vi "PreSequenceAcquisition.vi"(8 "error in (no error)":errorcluster, 10 "Acquisition Params":T1 {"Interval" min=0.0 max=99999.0; "Frames" min=0.0 max=5000.0; "ExposureMs" min=0.0 max=99999.0}, 11 "Camera_Prime95B in":refnum<class "Camera_Prime95B.lvclass">) -> (0 "error out":errorcluster, 3 "Camera_Prime95B out":refnum<class "Camera_Prime95B.lvclass">)   [LabVIEW 2020, in "Camera_Prime95B.lvlib" / "Camera_Prime95B.lvclass"]
uses:
  Camera_Prime95B.lvclass
  Acquisition Params.ctl
  Camera_Prime95B.lvclass/Camera_Prime95B.ctl
  D:/Daguan/Development/MMicroscopyAF/Model/Real Hardware/Camera_Prime95B/Camera_Prime95B/Dependencies/PVCamNET.dll
  Dependencies/PVCamNET.dll
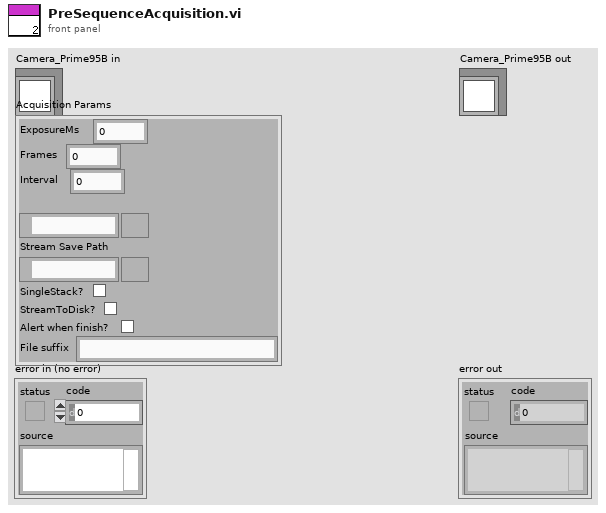
[diagram p1: front panel]
types:
  T1 = typedef "Camera_Prime95B.lvlib/Camera_Prime95B.lvclass/Acquisition Params.ctl" = cluster{"ExposureMs":dbl, "Frames":dbl, "Interval":dbl, "Save Path":path, "Stream Save Path":path, "SingleStack?":bool, "StreamToDisk?":bool, "Alert when finish?":bool, "File suffix":string}
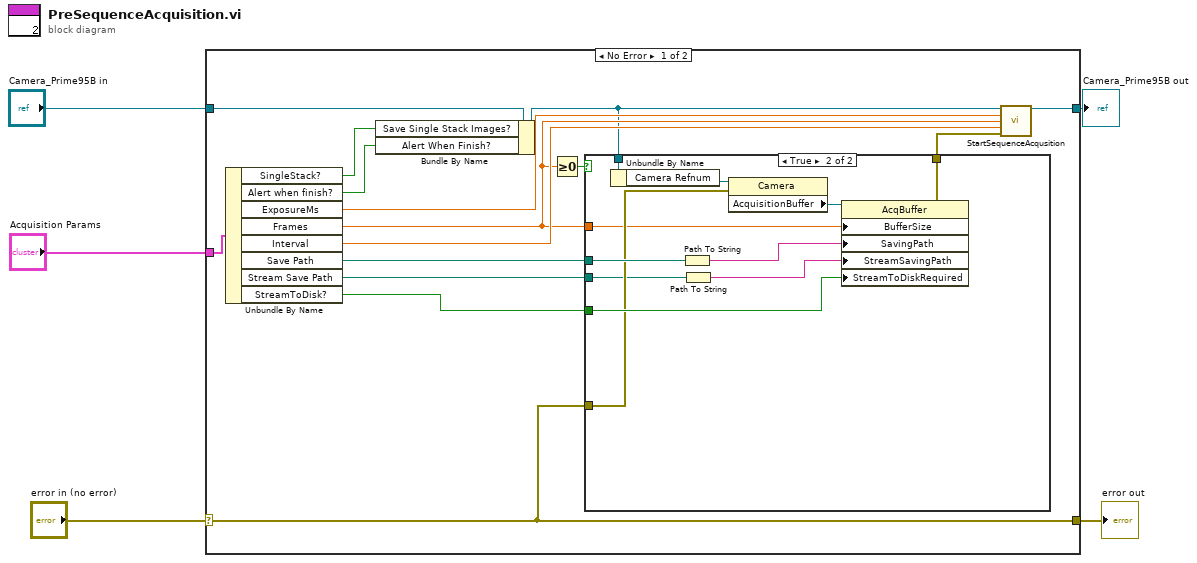
[diagram p0: block diagram]
diagram:
  n1 = case shown="No Error" "error in (no error)" {
    selector: "error in (no error)" -> [w12 w34]
    tunnel: [w12 w34] -> w4
    tunnel: [w19 w33] -> w2
    tunnel: "Camera_Prime95B in" -> [w14 w33]
    tunnel: "Acquisition Params" -> [w20 _]
    frame No Error {
      n2 = Unbundle By Name(w20) -> ("SingleStack?"=w6:bool, "Alert when finish?"=w7:bool, "ExposureMs"=w18:dbl, "Frames"=w9:dbl, "Interval"=w17:dbl, "Save Path"=w15:path, "Stream Save Path"=w10:path, "StreamToDisk?"=w11:bool)
      n3 = Bundle By Name(cluster=w14, "Save Single Stack Images?"=w6, "Alert When Finish?"=w7) -> (w8:refnum<class "Camera_Prime95B.lvclass">)
      n4 = Greater Or Equal To 0?(x=w9) -> (x >= 0?=w16:bool)
      n5 = case shown="True" w16 {
        tunnel: w15 -> [_ w28]
        tunnel: w8 -> [_ w32]
        tunnel: w11 -> [_ w29]
        tunnel: [w21 w27] -> w13
        tunnel: w12 -> [w21 w26]
        tunnel: w10 -> [_ w25]
        tunnel: w9 -> [_ w22]
        frame False {
        }
        frame True {
          n6 = Unbundle By Name(w32) -> ("Camera Refnum"=w31:refnum<k24>)
          n7 = Path To String(path=w28) -> (string=w23:string)
          n8 = Path To String(path=w25) -> (string=w24:string)
          n9 = property class="Camera"(reference=w31, error in=w26) -> ("AcquisitionBuffer"=w30:refnum<k24>)  [unwired: 2 out]
          n10 = property class="AcqBuffer"(reference=w30, "BufferSize"=w22, "SavingPath"=w23, "StreamSavingPath"=w24, "StreamToDiskRequired"=w29) -> (error out=w27:errorcluster)  [unwired: 1 in, 1 out]
        }
      }
      n11 = call-dynamic "StartSequenceAcqusition.vi"("Camera_Prime95B in"=w8, "Exposure"=w18, "Frames"=w9, "Interval"=w17, "error in (no error)"=w13) -> ("Camera_Prime95B out"=w19:refnum<class "Camera_Prime95B.lvclass">)  [unwired: 9 in, 1 out]
    }
    frame Error {
    }
  }
  "error out" <- w4
  "Camera_Prime95B out" <- w2
